vi "Calibração.vi"() -> ()   [LabVIEW 2016]
uses:
  <vilib>/University of Leeds/Kinesthesia Toolkit for Microsoft Kinect/_Polymorphic Close/Close-Skeleton and Video.vi
panel:
  out "XY Graph":cluster{"Wavenumber":dbl[], "Data":dbl[]}(graph)
  out "d.kinect":string caption="Distância percorrida pelo Kinect"
  out "d.sensor":string caption="Distância percorrida pelo Sensor"
  out "Array":string[](array[string])
  in  "select":u16(ring) items=["Samsung Galaxy J3 (2016)"]
  in  "refresh":bool
  out "calibração":u8(slide) scale=0.0..100.0
  in  "iniciar_calibração":bool
  in  "Ligar Acelerômetro":bool
  in  "Ligar Kinects":bool
  in  "Listbox":i32(listbox)
  # "Calibração do Kinect"
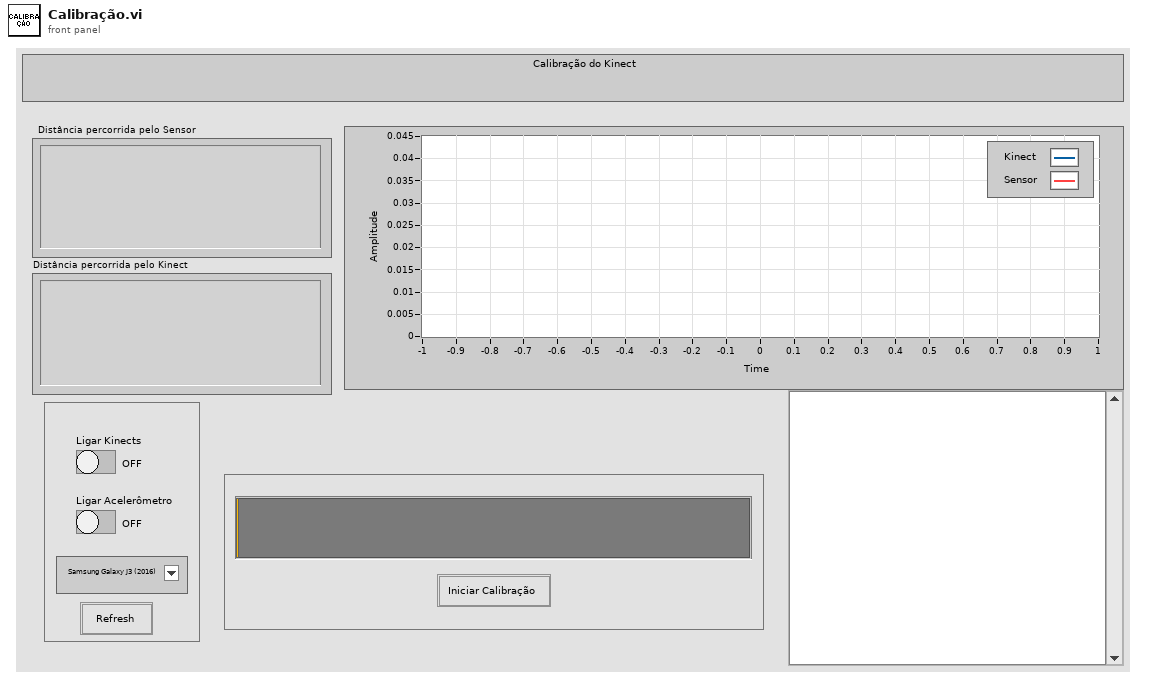
[diagram p1: front panel]
types:
  T1 = enum16{"Standard", "Buffered", "CRLF", "Immediate"}
  T2 = cluster{"reference out":refnum<k24>, "KinectSensors":refnum<k24>, "SkeletonStream":refnum<k24>, "ColorStream":refnum<k24>, refnum<k24>[], "get_Item":refnum<k24>}
  T3 = cluster{cluster{"reference out":refnum<k24>, "KinectSensors":refnum<k24>}, "get_Item":refnum<k24>}
  T4 = cluster{"Address":string, "Device Name":string}[]
  T5 = cluster{"channel":u16, "uuid":string, "service name":string, "service description":string}[]
  T6 = cluster{"channel":u16, "uuid":string, "service name":string, "service description":string}
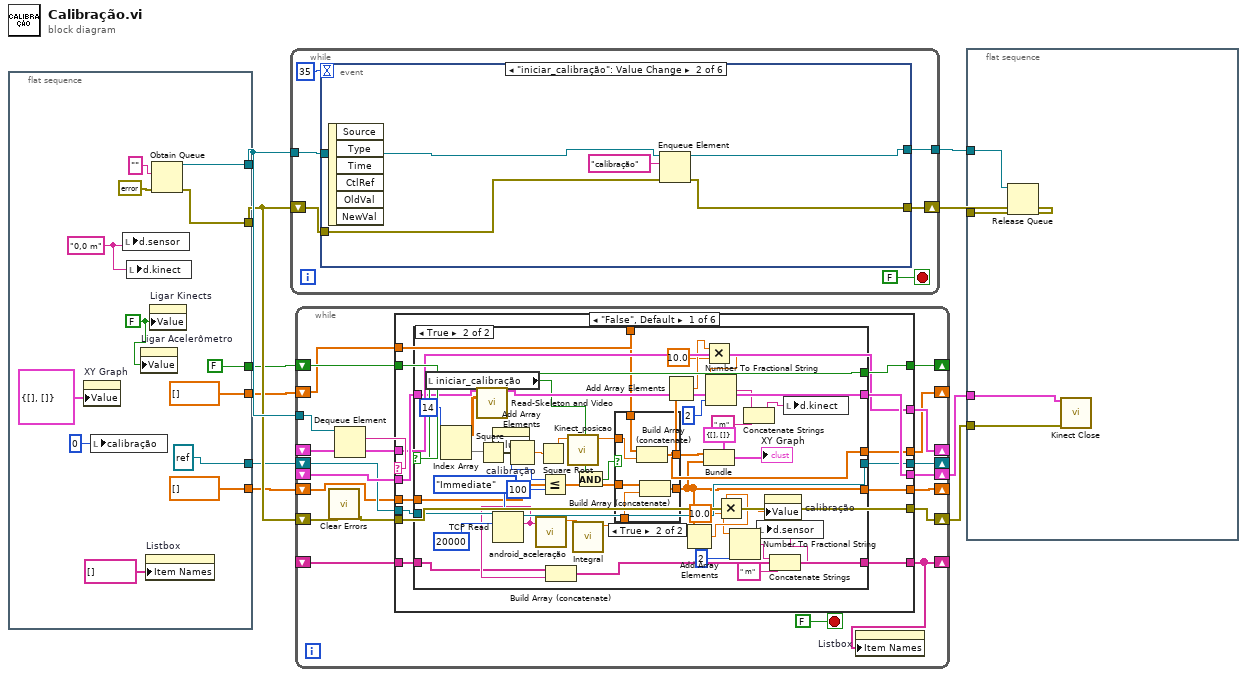
[diagram p0: block diagram]
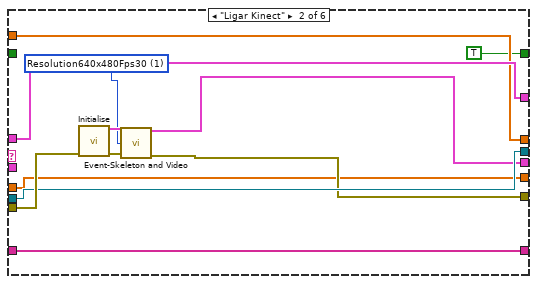
[diagram p4: hidden frame]
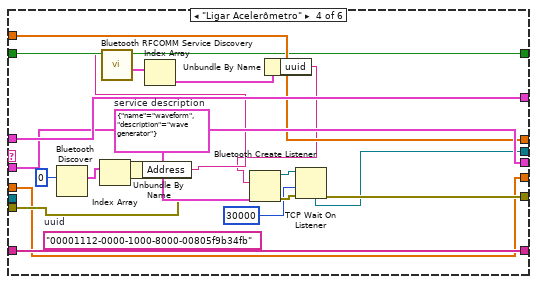
[diagram p6: hidden frame]
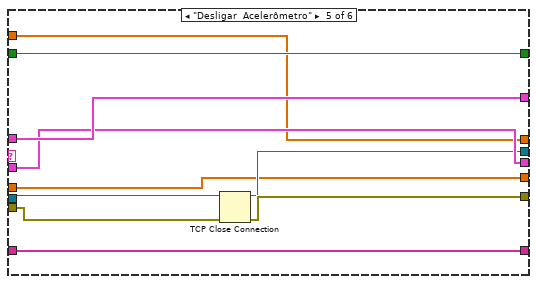
[diagram p7: hidden frame]
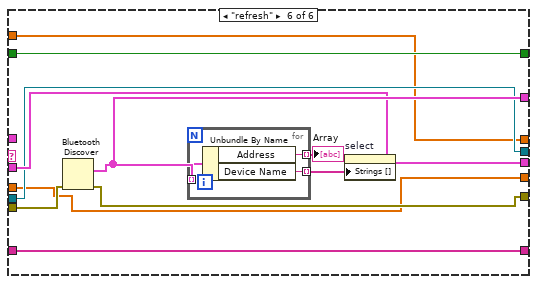
[diagram p8: hidden frame]
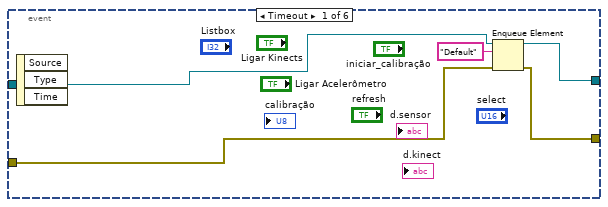
[diagram p9: hidden frame]
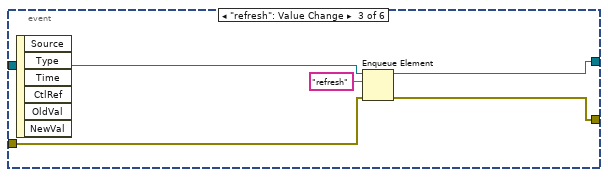
[diagram p10: hidden frame]
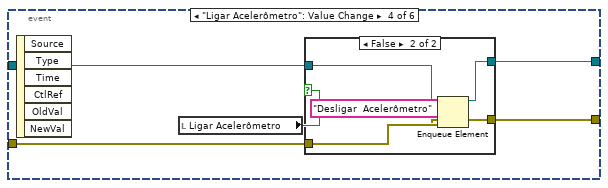
[diagram p11: hidden frame]
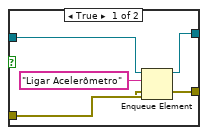
[diagram p12: hidden frame]
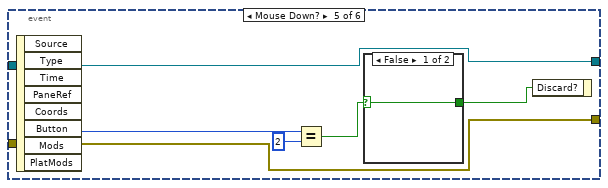
[diagram p13: hidden frame]
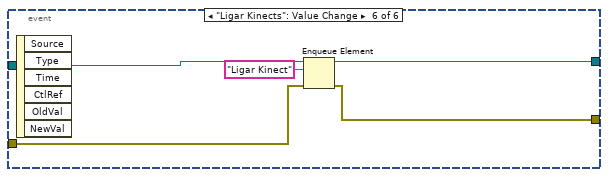
[diagram p15: hidden frame]
diagram:
  n1 = flat-sequence {
    tunnel: [w23] -> w10
    tunnel: [w21] -> w9
    tunnel: [dbl[] []] -> w5
    tunnel: [dbl[] []] -> w4
    tunnel: [refnum<k31> refnum ("connection ID")] -> w3
    tunnel: [FALSE] -> w2
    frame #0 {
      w14 = "0,0 m" ("d.sensor")
      w16 = FALSE ("Ligar Kinects")
      n2 = property on="XY Graph" class="XYGraph (strict)"("Value"=cluster{"Wavenumber":dbl[], "Data":dbl[]} {"Wavenumber"=[], "Data"=[]} ("XY Graph")) -> ()  [unwired: 2 in, 2 out]
      n3 = local write "calibração"(u8 0 ("calibração")) -> ()
      n4 = local write "d.sensor"(w14) -> ()
      n5 = local write "d.kinect"(w14) -> ()
      n6 = property on="Ligar Acelerômetro" class="Bool (strict)"("Value"=w16) -> ()  [unwired: 2 in, 2 out]
      n7 = property on="Listbox" class="LstBox (strict)"("Item Names"=string[] []) -> ()  [unwired: 2 in, 2 out]
      n8 = property on="Ligar Kinects" class="Bool (strict)"("Value"=w16) -> ()  [unwired: 2 in, 2 out]
      n9 = Obtain Queue(element data type="" ("name (unnamed)"), error in (no error)=errorcluster {"status"=FALSE, "code"=0, "source"=""} ("error constant")) -> (queue out=w23:refnum<queue>, error out=w21:errorcluster)  [unwired: 3 in, 1 out]
    }
  }
  n10 = while {
    tunnel: w10 -> [w28]
    shift-right: [w26] -> w8
    shift-left: w9 -> [w27]
    tunnel: [w25] -> w7
    stop <- FALSE stop-if-true
    n11 = event shown="[1] \"iniciar_calibração\": Value Change" {
      selector: _ -> [_ _ _ _ _ _]
      dyn-events: _ -> [_ _ _ _ _ _]
      timeout: 35 -> [_ _ _ _ _ _]
      tunnel: w28 -> [w31 w38 w40 w49 w61 w72]
      tunnel: w27 -> [w34 w37 w43 w47 w60 w71]
      tunnel: [w33 w36 w42 w46 w60 w70] -> w26
      tunnel: [w30 w35 w41 w48 w61 w68] -> w25
      event Timeout {
        n12 = event-data() -> ()  [unwired: 1 in, 3 out]
        n13 = Enqueue Element(queue=w31, element="Default", error in (no error)=w34) -> (queue out=w30:refnum<queue>, error out=w33:errorcluster)  [unwired: 1 in, 1 out]
      }
      event "iniciar_calibração": Value Change {
        n14 = event-data() -> ()  [unwired: 1 in, 6 out]
        n15 = Enqueue Element(queue=w38, element="calibração", error in (no error)=w37) -> (queue out=w35:refnum<queue>, error out=w36:errorcluster)  [unwired: 1 in, 1 out]
      }
      event "refresh": Value Change {
        n16 = event-data() -> ()  [unwired: 1 in, 6 out]
        n17 = Enqueue Element(queue=w40, element="refresh", error in (no error)=w43) -> (queue out=w41:refnum<queue>, error out=w42:errorcluster)  [unwired: 1 in, 1 out]
      }
      event "Ligar Acelerômetro": Value Change {
        n18 = event-data() -> ()  [unwired: 1 in, 6 out]
        n19 = local read "Ligar Acelerômetro"() -> (w45:bool)
        n20 = case shown="False" w45 {
          tunnel: w49 -> [w54 w59]
          tunnel: [w53 w58] -> w48
          tunnel: w47 -> [w51 w56]
          tunnel: [w50 w55] -> w46
          frame True {
            n21 = Enqueue Element(queue=w54, element="Ligar Acelerômetro", error in (no error)=w51) -> (queue out=w53:refnum<queue>, error out=w50:errorcluster)  [unwired: 1 in, 1 out]
          }
          frame False {
            n22 = Enqueue Element(queue=w59, element="Desligar  Acelerômetro", error in (no error)=w56) -> (queue out=w58:refnum<queue>, error out=w55:errorcluster)  [unwired: 1 in, 1 out]
          }
        }
      }
      event Mouse Down? {
        n23 = event-data() -> ("Button"=w65:u16)  [unwired: 1 in, 7 out]
        n24 = Equal?(x=w65, y=u16 2) -> (x = y?=w62:bool)
        n25 = case shown="False" w62 {
          selector: w62 -> [w66 w67]
          tunnel: [w66 w67] -> w63
          frame False {
          }
          frame True {
          }
        }
        n26 = event-data("Discard?"=w63) -> ()  [unwired: 1 in, 1 out]
      }
      event "Ligar Kinects": Value Change {
        n27 = event-data() -> ()  [unwired: 1 in, 6 out]
        n28 = Enqueue Element(queue=w72, element="Ligar Kinect", error in (no error)=w71) -> (queue out=w68:refnum<queue>, error out=w70:errorcluster)  [unwired: 1 in, 1 out]
      }
    }
  }
  n29 = while {
    tunnel: w10 -> [w91]
    shift-right: [w89] -> w1
    shift-left: w9 -> [w79]
    shift-right: [w88] -> _
    shift-left: _ -> [w87]
    shift-right: [w85] -> _
    shift-left: w2 -> [w84]
    shift-right: [w83] -> w6
    shift-left: _ -> [w82]
    shift-right: [w86] -> _
    shift-left: w3 -> [w81]
    shift-right: [w73] -> _
    shift-left: w4 -> [w78]
    shift-right: [w76] -> _
    shift-left: w5 -> [w77]
    shift-right: [w74] -> _
    shift-left: _ -> [w75]
    stop <- FALSE stop-if-true
    n30 = call <vilib>:"Clear Errors.vi"("error in (no error)"=w79) -> ("error out"=w80:errorcluster)  [unwired: 5 in, 1 out]
    n31 = Dequeue Element(queue=w91) -> (element=w90:string)  [unwired: 2 in, 3 out]
    n32 = case shown="\"False\", Default" w90 {
      tunnel: w80 -> [w106 w176 w182 w193 w210 w219]
      tunnel: [w106 w169 w182 w199 w209 w220] -> w89
      tunnel: [w100 w175 w184 w204 w214 w225] -> w88
      tunnel: w87 -> [w100 w175 w184 w204 w214 _]
      tunnel: [w99 w174 w181 w196 w208 w222] -> w86
      tunnel: [w104 TRUE w179 w194 w212 w224] -> w85
      tunnel: w84 -> [w105 _ w179 w194 w212 w224]
      tunnel: [w101 w171 w183 w203 w213 w223] -> w83
      tunnel: w82 -> [w103 _ w183 w203 w213 w223]
      tunnel: w81 -> [w102 w174 w181 _ w211 w222]
      tunnel: w78 -> [w98 w165 w177 w185 w205 w215]
      tunnel: w77 -> [w97 w168 w180 w198 w207 w218]
      tunnel: [w96 w168 w180 w198 w207 w218] -> w76
      tunnel: w75 -> [w95 w166 w178 w195 w206 w216]
      tunnel: [w94 w166 w178 w195 w206 w216] -> w74
      tunnel: [w93 w165 w177 w185 w205 w215] -> w73
      frame "False", Default {
        n33 = case shown="True" w105 {
          selector: w105 -> [w112 w156]
          tunnel: [w112 w156] -> w104
          tunnel: w103 -> [w111 w153]
          tunnel: w102 -> [w110 w155]
          tunnel: [w111 w152] -> w101
          tunnel: [w110 w154] -> w99
          tunnel: w98 -> [w107 w139]
          tunnel: w97 -> [w109 w143]
          tunnel: [w109 w133] -> w96
          tunnel: w95 -> [w108 w141]
          tunnel: [w108 w140] -> w94
          tunnel: [w107 w130] -> w93
          frame False {
          }
          frame True {
            n34 = local read "iniciar_calibração"() -> (w126:bool)
            n35 = call <vilib>:"Read-Skeleton and Video.vi"("Kinect References in"=w153) -> ("Primary Skeleton Array"=w148:dbl[][], "Kinect References out"=w152:T2)  [unwired: 10 in, 3 out]
            n36 = Index Array(array=w148, index (row)=14) -> (element=w145:dbl[])  [unwired: 1 in]
            n37 = Square(x=w145) -> (x^2=w146:dbl[])
            n38 = property on="calibração" class="Slide (strict)"() -> ("Value"=w129:u8)  [unwired: 2 in, 2 out]
            n39 = TCP Read(connection ID=w155, bytes to read=20000, 7:T1."Immediate" ("mode (standard)")) -> (connection ID out=w154:refnum<k31>, data out=w142:string)  [unwired: 2 in, 1 out]
            n40 = Add Array Elements(numeric array=w146) -> (sum=w144:dbl)
            n41 = call "android_aceleração.vi"("Dados Sensor"=w142) -> ("Aceleração"=w138:dbl)  [unwired: 10 in]
            n42 = Square Root(x=w144) -> (sqrt(x)=w135:dbl)
            n43 = Less Or Equal?(x=w129, y=u8 100) -> (x <= y?=w127:bool)
            n44 = Build Array (concatenate)(w141, w142) -> (w140:string[])
            n45 = call "Kinect_posicao.vi"("dado"=w135) -> ("Old Value"=w134:dbl)  [unwired: 10 in]
            n46 = call "Integral.vi"("Aceleração atual"=w138) -> ("Posição"=w131:dbl)  [unwired: 9 in, 1 out]
            n47 = And(x=w126, y=w127) -> (x .and. y?=w125:bool)
            n48 = case shown="True" w125 {
              tunnel: w143 -> [w158 w164]
              tunnel: w139 -> [w157 w163]
              tunnel: [w157 w162] -> w130
              tunnel: w134 -> [_ w161]
              tunnel: [w158 w160] -> w133
              tunnel: w131 -> [_ w159]
              frame False {
              }
              frame True {
                n49 = Build Array (concatenate)(w164, w161) -> (w160:dbl[])
                n50 = Build Array (concatenate)(w163, w159) -> (w162:dbl[])
              }
            }
            n51 = Add Array Elements(numeric array=w133) -> (sum=w115:dbl)
            n52 = Add Array Elements(numeric array=w130) -> (sum=w117:dbl)
            n53 = Multiply(x=w115, y=10.0) -> (x*y=w113:dbl)
            n54 = Bundle(cluster=cluster{"Wavenumber":dbl[], "Data":dbl[]} {"Wavenumber"=[], "Data"=[]} ("Spectrum"), "Wavenumber"=w133, "Data"=w130) -> (→"XY Graph":cluster{"Wavenumber":dbl[], "Data":dbl[]})
            n55 = Number To Fractional String(number=w113, precision (6)=i16 2) -> (F-format string=w120:string)  [unwired: 2 in]
            n56 = Multiply(x=w117, y=10.0) -> (x*y=w116:dbl)
            n57 = Number To Fractional String(number=w116, precision (6)=i16 2) -> (F-format string=w123:string)  [unwired: 2 in]
            n58 = Concatenate Strings(w120, " m" ("string")) -> (w119:string)
            n59 = property on="calibração" class="Slide (strict)"("Value"=w116) -> ()  [unwired: 2 in, 2 out]
            n60 = Concatenate Strings(w123, " m" ("string")) -> (w124:string)
            n61 = local write "d.sensor"(w124) -> ()
            n62 = local write "d.kinect"(w119) -> ()
          }
        }
      }
      frame "Ligar Kinect" {
        w170 = 1 items=["Undefined", "Resolution640x480Fps30", "Resolution320x240Fps30", "Resolution80x60Fps30"] ("Depth Stream Format")
        n63 = call <vilib>:"Initialise.vi"("error in (no error)"=w176) -> ("Kinect References out"=w173:T3, "error out"=w172:errorcluster)  [unwired: 13 in]
        n64 = call <vilib>:"Event-Skeleton and Video.vi"("Kinect References in"=w173, "RGB Stream Format"=w170, "error in"=w172) -> ("Kinect References out"=w171:T2, "error out"=w169:errorcluster)  [unwired: 11 in]
      }
      frame "calibração" {
      }
      frame "Ligar Acelerômetro" {
        w201 = cluster{"name":string, "description":string} {"name"="waveform", "description"="wave generator"}  # service description
        (unwired) "00001112-0000-1000-8000-00805f9b34fb"  # uuid
        n65 = Bluetooth Discover(10:0 ("time limit ms (10000)")) -> (2:w189:T4)  [unwired: 1 in, 2 out]
        n66 = Index Array(array=w189) -> (element=w188:cluster{"Address":string, "Device Name":string})  [unwired: 1 in]
        n67 = Unbundle By Name(w188) -> ("Address"=w187:string)
        n68 = call <vilib>:"Bluetooth RFCOMM Service Discovery.vi"("address in"=w187) -> ("service list"=w192:T5)  [unwired: 3 in, 3 out]
        n69 = Index Array(array=w192) -> (element=w191:T6)  [unwired: 1 in]
        n70 = Unbundle By Name(w191) -> ("uuid"=w186:string)
        n71 = Bluetooth Create Listener(6:w201, 8:w193, 10:w186) -> (0:w202:errorcluster, 3:w200:refnum<k31>)  [unwired: 2 out]
        n72 = TCP Wait On Listener(8:w202, 9:30000 ("timeout ms (wait forever: -1)"), 11:w200) -> (0:w199:errorcluster, 4:w196:refnum<k31>)  [unwired: 4 out]
      }
      frame "Desligar  Acelerômetro" {
        n73 = TCP Close Connection(connection ID=w211, error in (no error)=w210) -> (connection ID out=w208:refnum<k31>, error out=w209:errorcluster)  [unwired: 1 in]
      }
      frame "refresh" {
        n74 = Bluetooth Discover(8:w219) -> (0:w220:errorcluster, 2:w225:T4)  [unwired: 1 in, 1 out]
        n75 = for {
          tunnel: w225 -> [w228] mode=indexing
          tunnel: [w227] -> w221 mode=indexing
          tunnel: [w226] -> w217 mode=indexing
          n76 = Unbundle By Name(w228) -> ("Address"=w226:string, "Device Name"=w227:string)
        }
        "Array" <- w217
        n77 = property on="select" class="Ring (strict)"("Strings []"=w221) -> ()  [unwired: 2 in, 2 out]
      }
    }
    n78 = property on="Listbox" class="LstBox (strict)"("Item Names"=w74) -> ()  [unwired: 2 in, 2 out]
  }
  n79 = flat-sequence {
    tunnel: w8 -> [w232]
    tunnel: w7 -> [w231]
    tunnel: w6 -> [w230]
    tunnel: w1 -> [w229]
    frame #0 {
      n80 = Release Queue(queue=w231, error in (no error)=w232) -> ()  [unwired: 1 in, 3 out]
      n81 = call-poly <vilib>:"Kinect Close.vi"("Kinect References in"=w230, "error in"=w229) -> ()  [unwired: 13 in, 1 out]
    }
  }
